vi "Relative Standard Deviation for one dimensional Array.vi"(10 "Input Array":dbl[](array[numeric])) -> (0 "Min Value":dbl, 1 "Max Value":dbl, 2 "mean":dbl format="%0.2f", 3 "Relative Standard Deviation":dbl)   [LabVIEW 2016]
uses:
  <vilib>/Analysis/baseanly.llb/Mean (DBL).vi
  <vilib>/Analysis/NI_AALBase.lvlib
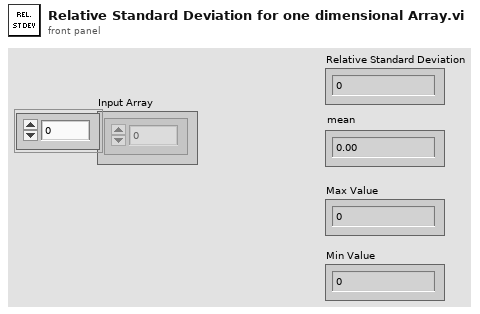
[diagram p1: front panel]
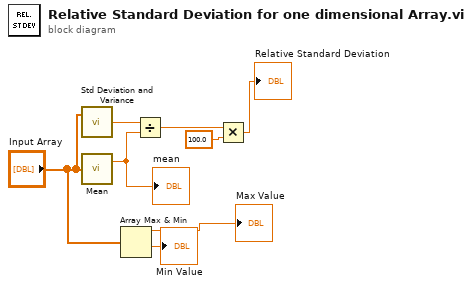
[diagram p0: block diagram]
diagram:
  n1 = call <vilib>:"Std Deviation and Variance.vi"("X"="Input Array") -> ("standard deviation"=w5:dbl)  [unwired: 1 in, 2 out]
  n2 = call-poly <vilib>:"Mean.vi"("X"="Input Array") -> ("mean"=w4:dbl)  [unwired: 1 out]
  "mean" <- w4
  n3 = Array Max & Min(array="Input Array") -> (max value=→"Max Value":dbl, min value=→"Min Value":dbl)  [unwired: 2 out]
  n4 = Divide(x=w5, y=w4) -> (x/y=w6:dbl)
  n5 = Multiply(x=w6, y=100.0) -> (x*y=→"Relative Standard Deviation":dbl)
